vi "MCL Sort By Column.vi"(8 "error in (no error)":errorcluster, 11 "CtlRef":refnum<vi>) -> (0 "error out":errorcluster, 3 "CtlRef out":refnum<vi>)   [LabVIEW 2019, in "GUI.lvlib"]
doc: "This VI sorts a multicolumn listbox when you click a column header. Click a column header once to sort that column in ascending order. Click the header again to sort the column in descending order. The VI reorders all other columns to maintain row integrity. You can wire a multicolumn listbox control reference to this VI."
uses:
  GUI.lvlib
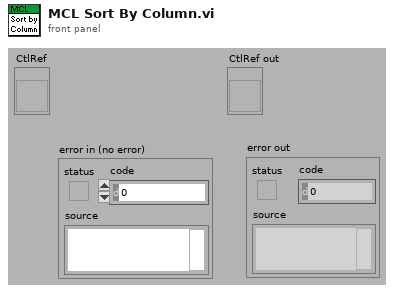
[diagram p1: front panel]
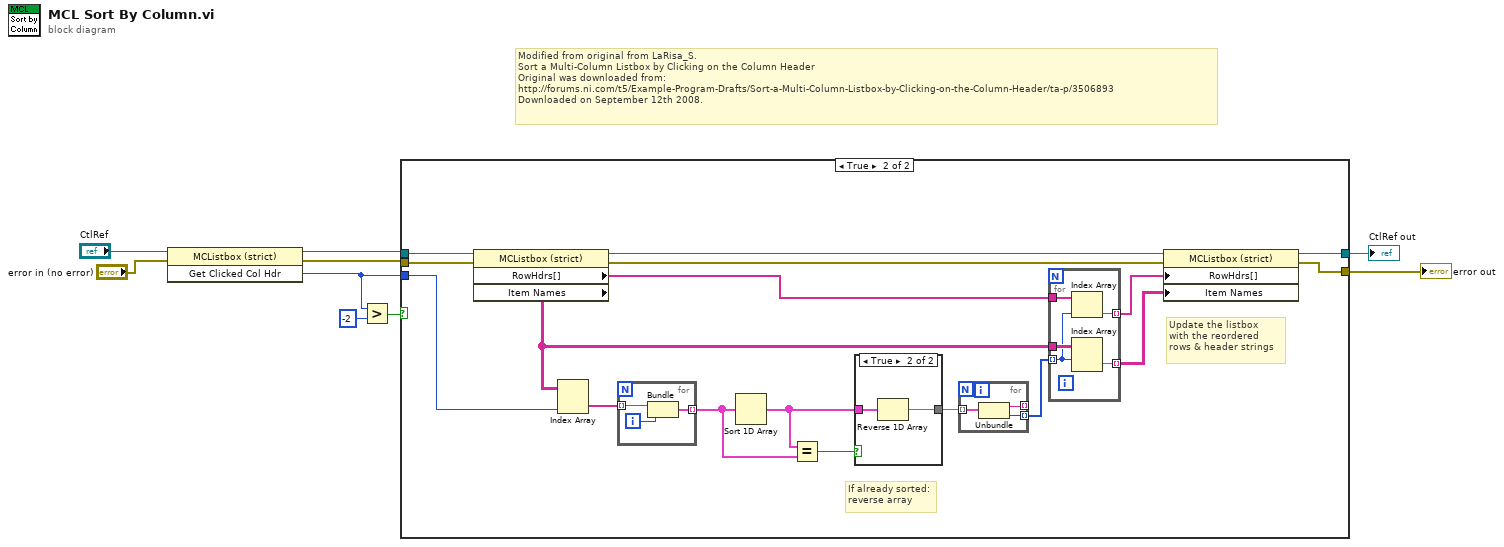
[diagram p0: block diagram]
diagram:
  # "Modified from original from LaRisa_S.\nSort a Multi-Column Listbox by Clicking on the Column Header\nOriginal was downloaded from:\nhttp://forums.ni.com/t5/Example-Program-Drafts/Sort-a-Multi-Column-Listbox-by-Clicking-on-the-Column-Header/ta-p/3506893\nDownloaded on September 12th 2008."
  n1 = invoke class="MCListbox (strict)" method="Get Clicked Col Hdr"(reference="CtlRef", error in="error in (no error)") -> (reference out=w4:refnum<vi>, error out=w6:errorcluster, "Get Clicked Column Header"=w5:i32)  [unwired: 1 in]
  n2 = Greater?(x=w5, y=-2) -> (0:w7:bool)
  n3 = case shown="True" w7 {
    tunnel: w5 -> [_ w28]
    tunnel: w6 -> [w11 w26]
    tunnel: w4 -> [w10 w27]
    tunnel: [w11 w21] -> w9
    tunnel: [w10 w20] -> w1
    frame False {
    }
    frame True {
      # "If already sorted:\nreverse array"
      # "Update the listbox\nwith the reordered\nrows & header strings"
      n4 = property class="MCListbox (strict)"(reference=w27, error in=w26) -> (reference out=w22:refnum<vi>, error out=w23:errorcluster, "RowHdrs[]"=w13:string[], "Item Names"=w25:string[][])
      n5 = Index Array(array=w25, index (col)=w28) -> (element=w16:string[])  [unwired: 1 in]
      n6 = for {
        tunnel: w16 -> [w31] mode=indexing
        tunnel: [w29] -> w15 mode=indexing
        i -> [w30]
        n7 = Bundle(w31, w30) -> (w29:cluster{string, i32})  [unwired: 1 out]
      }
      n8 = Sort 1D Array(array=w15) -> (sorted array=w18:cluster{string, i32}[])
      n9 = Equal?(x=w18, y=w15) -> (x = y?=w19:bool)
      n10 = case shown="True" w19 {
        tunnel: w18 -> [w32 w34]
        tunnel: [w32 w33] -> w17
        frame False {
        }
        frame True {
          n11 = Reverse 1D Array(array=w34) -> (reversed array=w33:cluster{string, i32}[])
        }
      }
      n12 = for {
        tunnel: w17 -> [w37] mode=indexing
        tunnel: [w36] -> _ mode=indexing
        tunnel: [w35] -> w14 mode=indexing
        n13 = Unbundle(w37) -> (w36:string, w35:i32)
      }
      n14 = for {
        tunnel: w14 -> [w39] mode=indexing
        tunnel: w25 -> [w42]
        tunnel: [w41] -> w24 mode=indexing
        tunnel: w13 -> [w40]
        tunnel: [w38] -> w12 mode=indexing
        n15 = Index Array(array=w40, index=w39) -> (element=w38:string)
        n16 = Index Array(array=w42, index (row)=w39) -> (element=w41:string[])  [unwired: 1 in]
      }
      n17 = property class="MCListbox (strict)"(reference=w22, error in=w23, "RowHdrs[]"=w12, "Item Names"=w24) -> (reference out=w20:refnum<vi>, error out=w21:errorcluster)
    }
  }
  "error out" <- w9
  "CtlRef out" <- w1
